vi "Main.vi"() -> ()   [LabVIEW 2021]
doc: "This template is for the Queued Message Handler design pattern.\n\nThe Event Handling Loop generates messages based on user interface actions.\n\nThe Message Handling Loop processes messages generated by the Event Handling Loop, or by other messages. The messages are string values, so new messages can be added easily to the Message Cases case structure in the Message Handling Loop. Each message cluster can also provide an optional value for Message Data, which is a variant that can be converted to whatever message-specific data is required."
uses:
  controls/UI Data.ctl
  support/Message Queue/Enqueue Message (Single).vi
  <vilib>/Analysis/3filter.llb/Butterworth Filter (DBL).vi
  <vilib>/Utility/error.llb/Error Cluster From Error Code.vi
  <vilib>/ErrorRing/Error Ring.xnode
  support/Message Queue/Message Queue.lvlib
  support/User Event - Stop/User Event - Stop.lvlib
  <vilib>/Analysis/NI_AALBase.lvlib
panel:
  in  "Engineering Mode":bool
  out "error out":errorcluster
  in  "Stop NanoJ":bool
  in  "Start NanoJ":bool
  out "Torque % of Max":dbl[](graph)
  in  "Read Torque":bool
  out "Motor Status":T1
  in  "Check Max Motor Current":bool
  out "Write":T2
  in  "Apply Speed":bool
  out "User Event":bool
  out "Actual Speed RPM":dbl(knob) scale=-110.0..110.0
  in  "Set Speed RPM":i32(knob) min=-60 max=60 scale=-60.0..60.0
  in  "Max Torque Nm":dbl=3.0 format="%.2f"
  out "Torque Nm":dbl
  out "Motor Current mA":dbl
  out "Max Motor Current mA":dbl
  out "Closed Loop Available":bool
  out "Motor Initialized":bool
  out "Torque\n%":dbl format="%.2f"
  in  "Halt Motor":bool
  in  "ComPort":refnum<visa-resource-name>="COM15"
  out "Program State":string
  in  "Start Motor":bool
  in  "Exit Program":bool
  # "<- Input max rated torque\nfor motor at Max Current Setting:"
  # "Current Motor Torque"
  # "Motor Current Draw"
  # "Set Speed Here \nthen click Apply\nto update Motor\nto new Velocity"
  # "Torque as percentage \nof Max Torque"
  # "Speed Value Read\nfrom Motor Memory"
  # "Restart the Motor Firmware\n(Hardware) Speed Controller\n(Disables LabVIEW Control)"
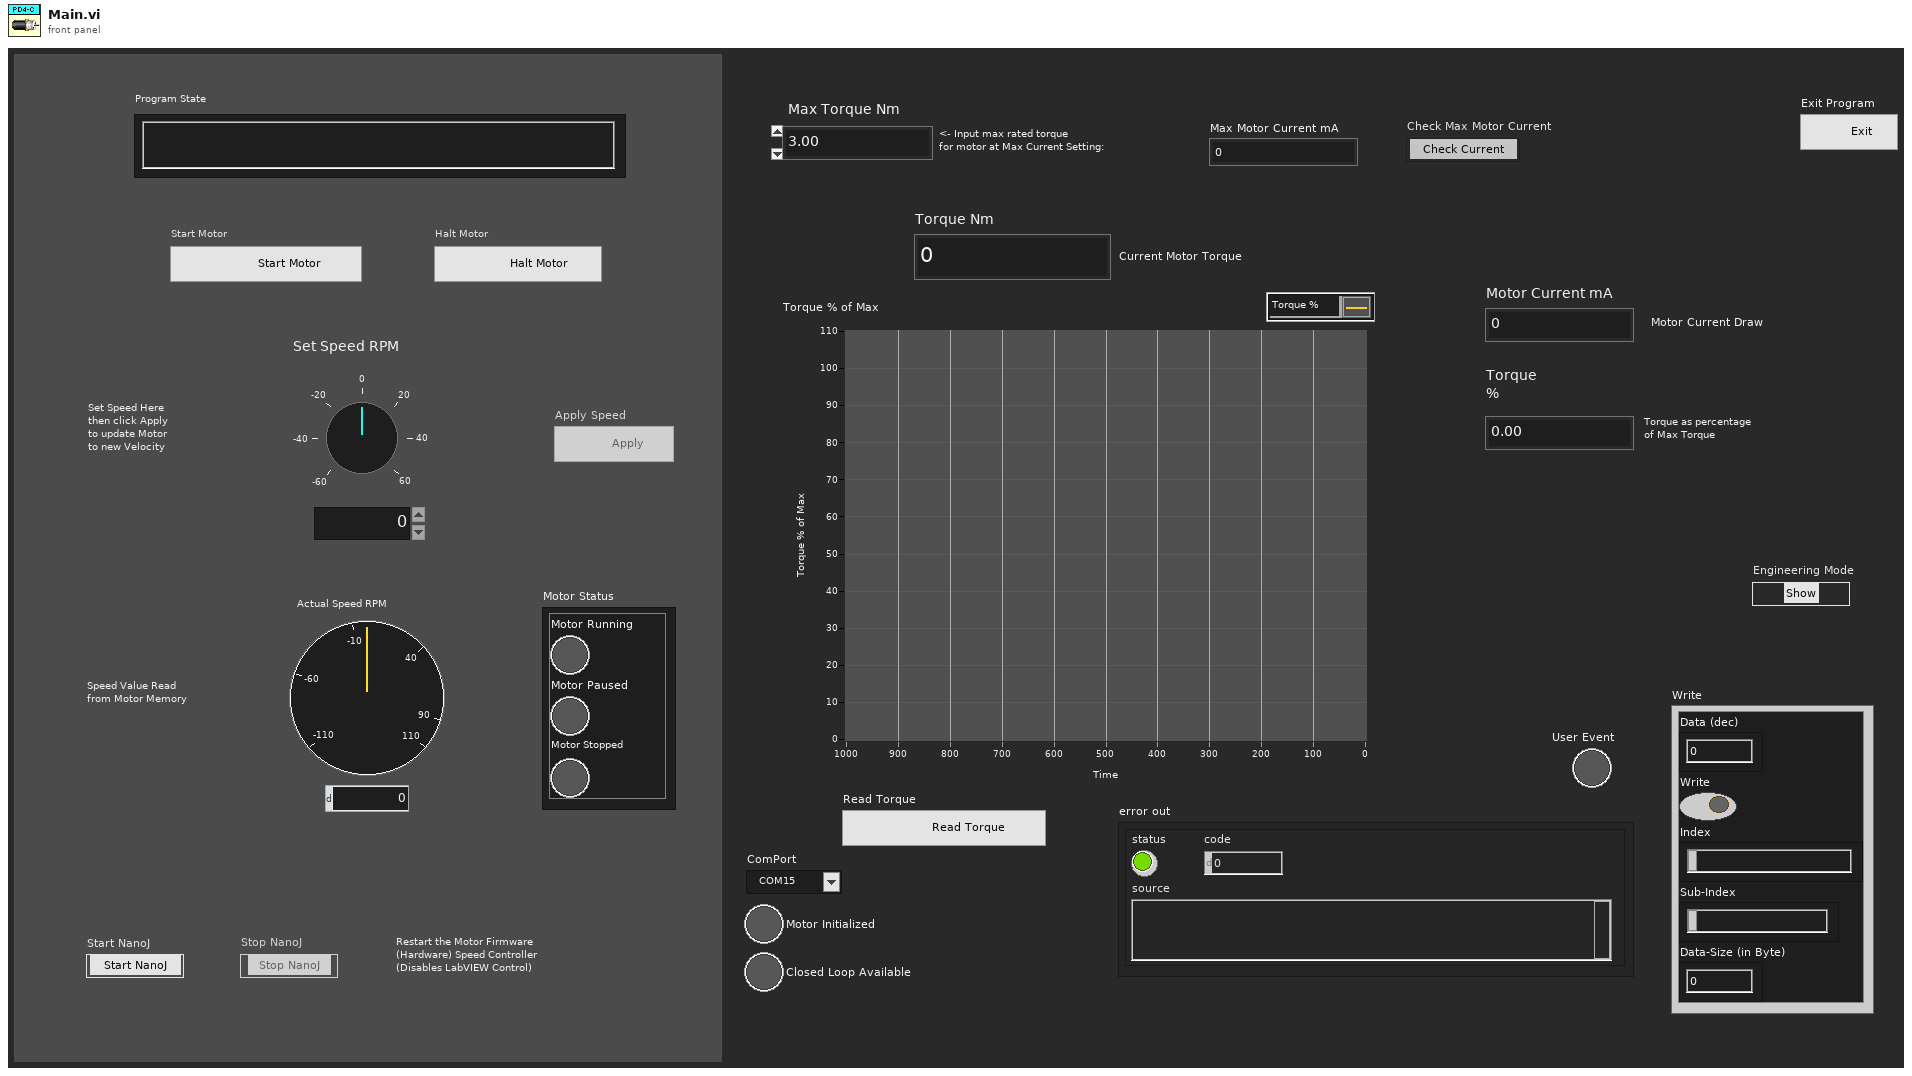
[diagram p1: front panel]
types:
  T1 = cluster{"Motor Running":bool, "Motor Paused":bool, "Motor Stopped":bool}
  T2 = cluster{"Data (dec)":i32, "Write":bool, "Index":string, "Sub-Index":string, "Data-Size (in Byte)":u8}
  T3 = typedef "UI Data.ctl" = cluster{"Data Display Ref":refnum<vi>, "Exit Button Ref":refnum<vi>, "VISA resource name":refnum<visa-resource-name>, "Write":cluster{"Data (dec)":i32, bool, "Index":string, "Sub-Index":string, "Data-Size (in Byte)":u8}, "Next State":string, "Data":i32}
  T4 = typedef "Message Queue.lvlib/All Message Queues.ctl" = cluster{"UI":refnum<queue>}
  T5 = enum8{"Enabled", "Disabled", "Disabled and Grayed Out"}
  T6 = cluster{"Motor Paused":bool, "Motor Running":bool, "Motor Stopped":bool}
  T7 = cluster{"Data (dec)":i32, bool, "Index":string, "Sub-Index":string, "Data-Size (in Byte)":u8}
  T8 = cluster{"Index":string, "Sub-Index":string, "Data-Size (in Byte)":u8, bool}
  T9 = cluster{"Motor Stopped":bool, "Motor Running":bool, "Motor Paused":bool}
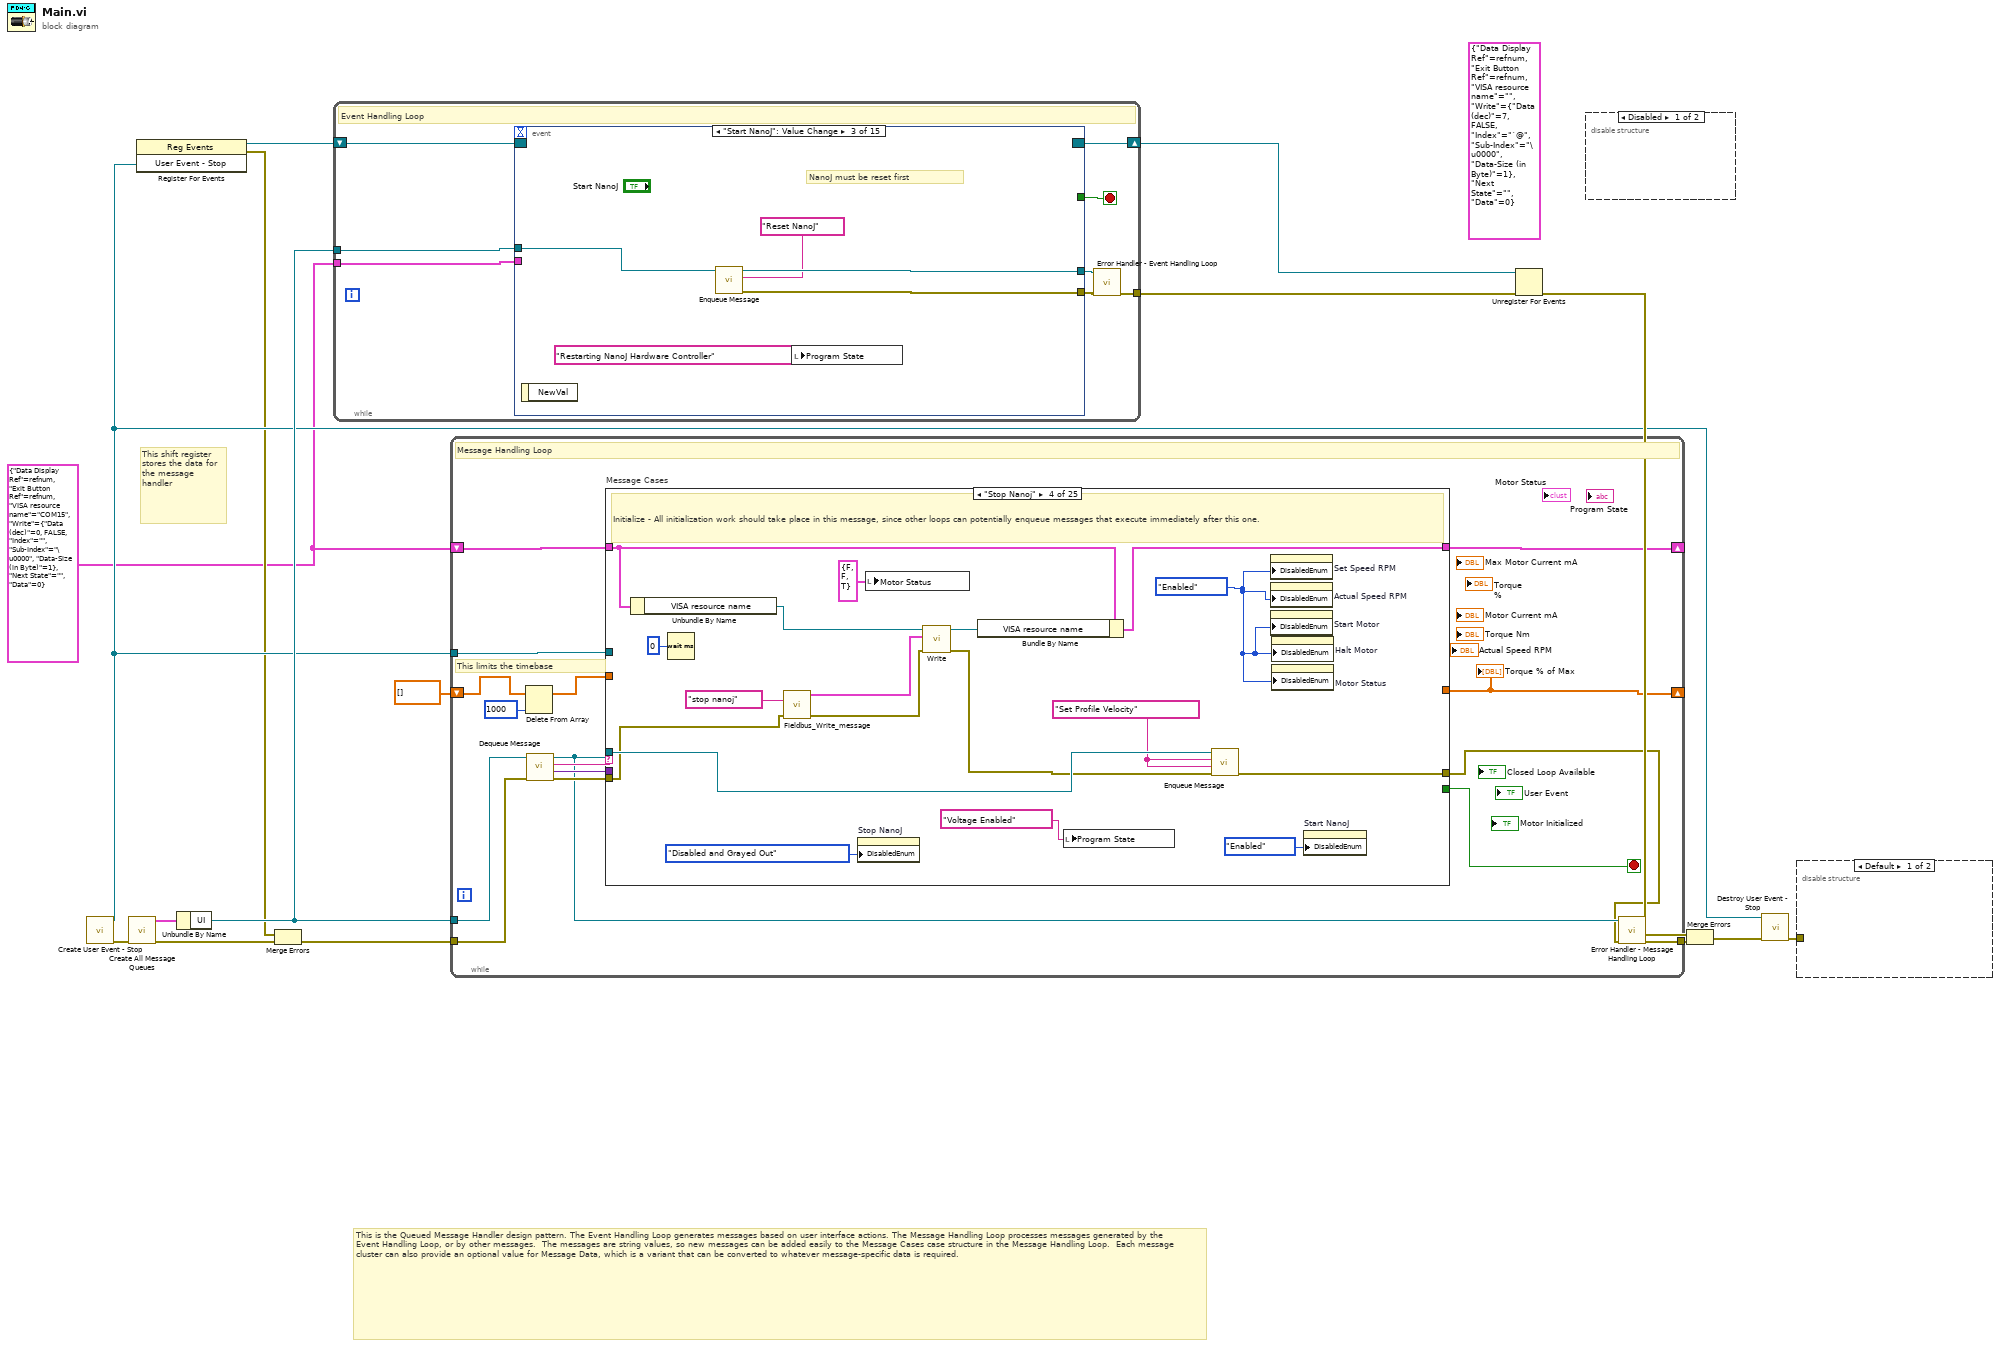
[diagram p0: block diagram]
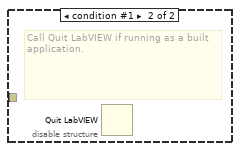
[diagram p3: hidden frame]
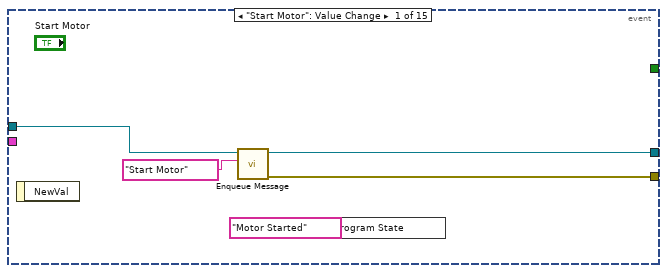
[diagram p4: hidden frame]
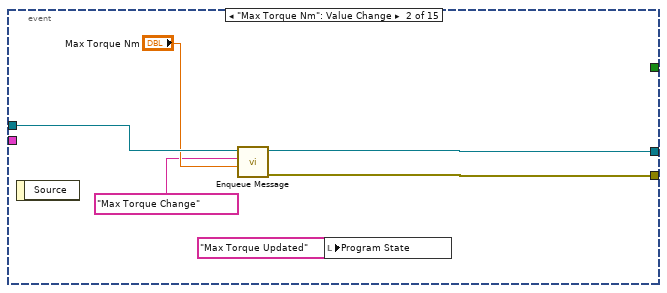
[diagram p5: hidden frame]
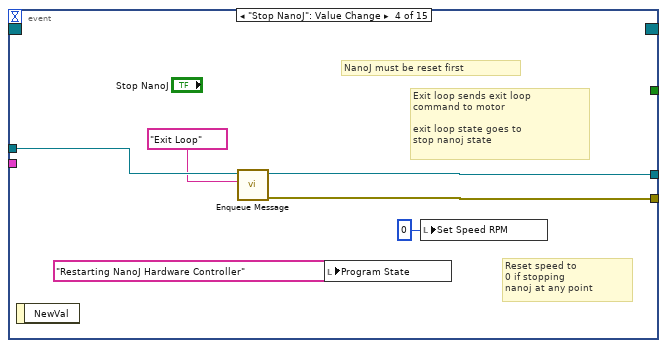
[diagram p6: hidden frame]
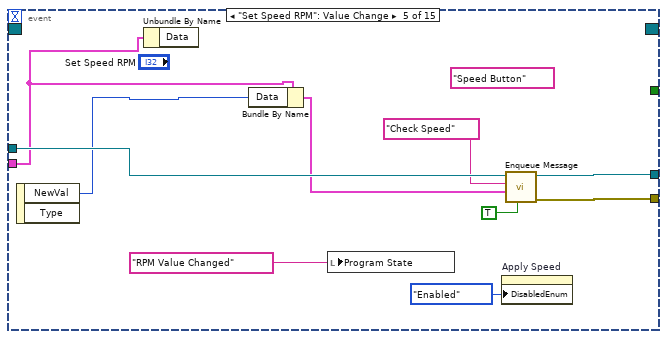
[diagram p7: hidden frame]
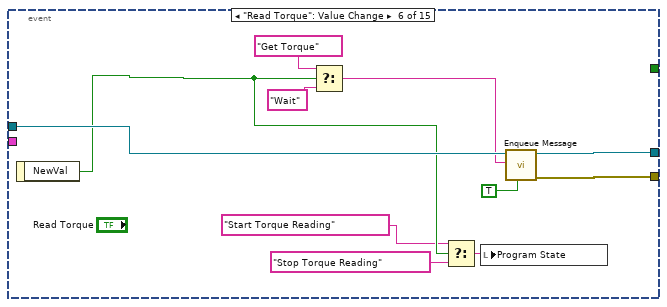
[diagram p8: hidden frame]
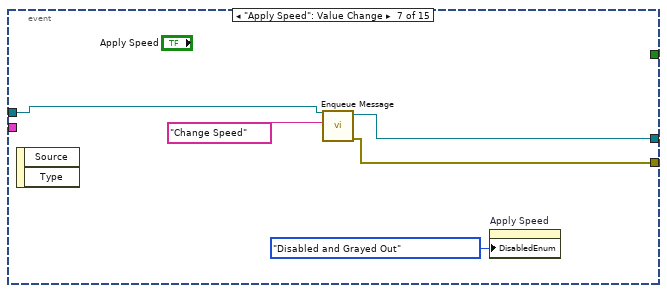
[diagram p9: hidden frame]
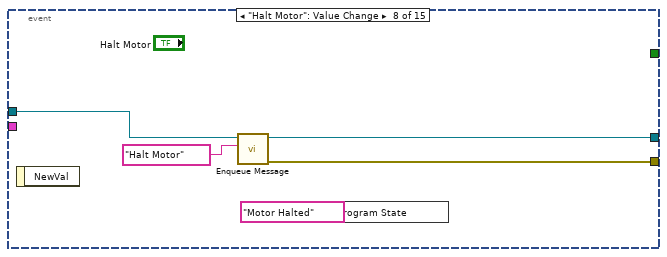
[diagram p10: hidden frame]
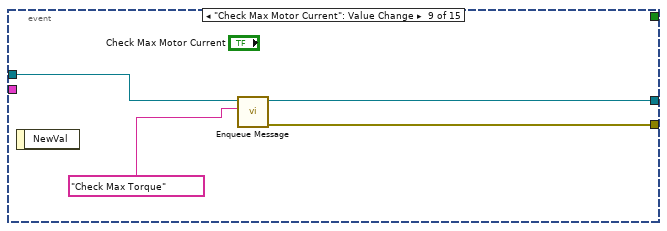
[diagram p11: hidden frame]
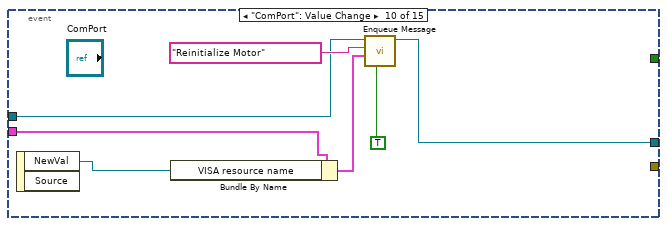
[diagram p12: hidden frame]
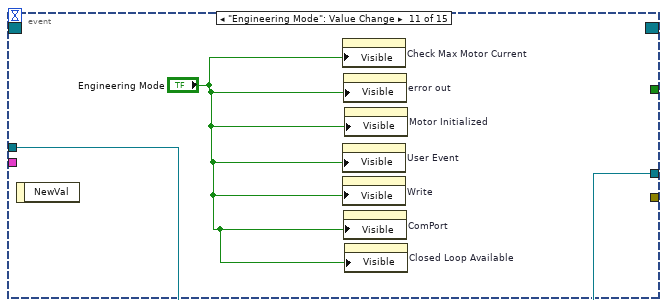
[diagram p13: hidden frame]
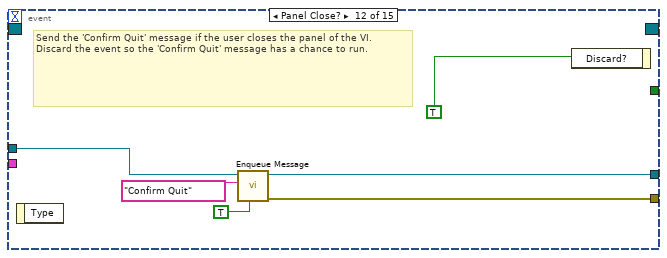
[diagram p14: hidden frame]
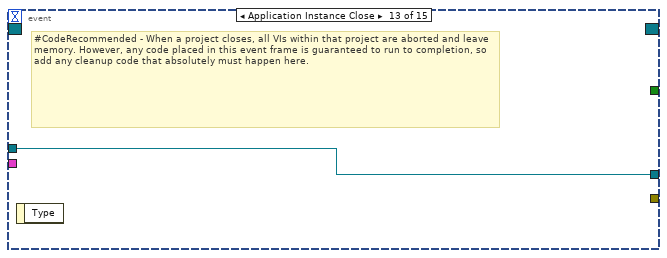
[diagram p15: hidden frame]
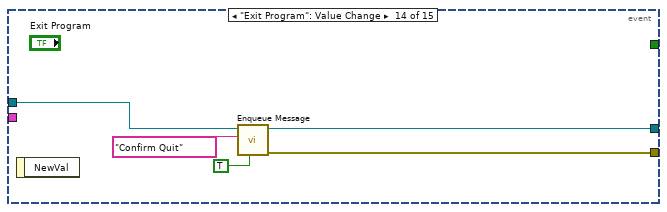
[diagram p16: hidden frame]
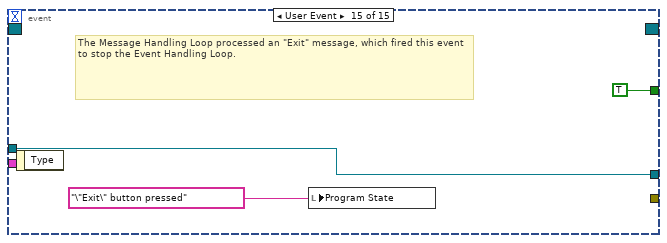
[diagram p17: hidden frame]
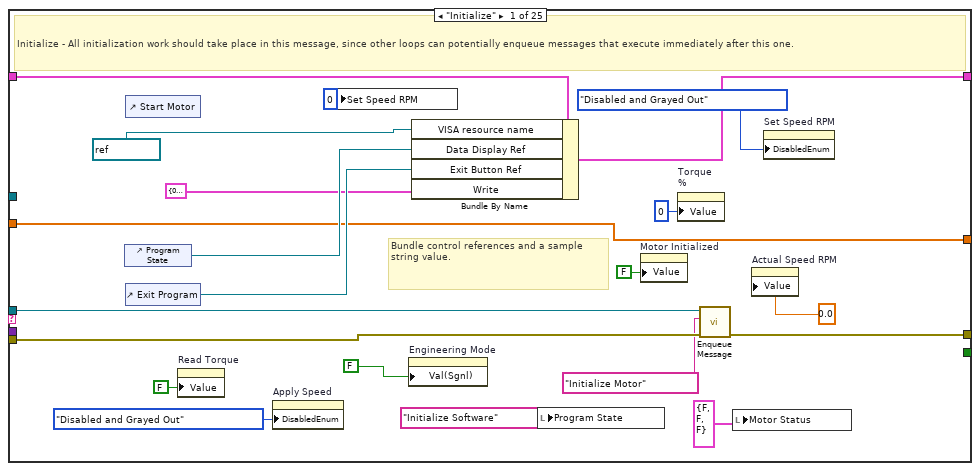
[diagram p18: hidden frame]
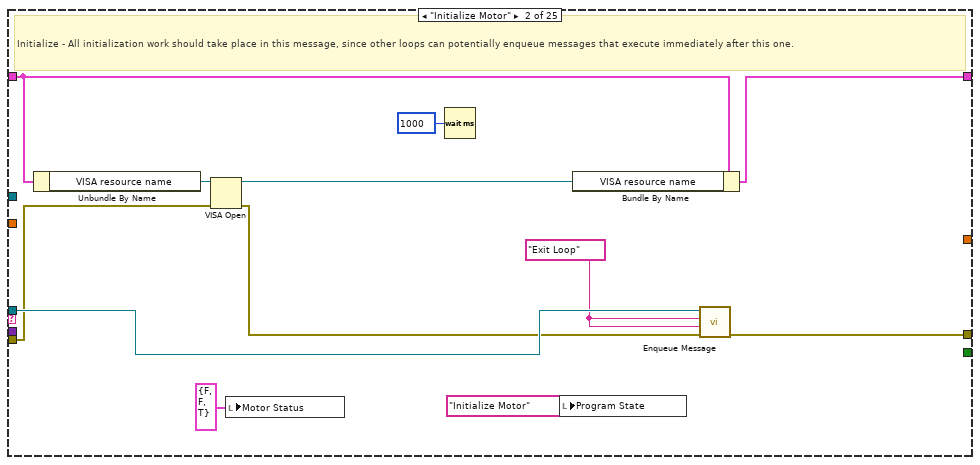
[diagram p19: hidden frame]
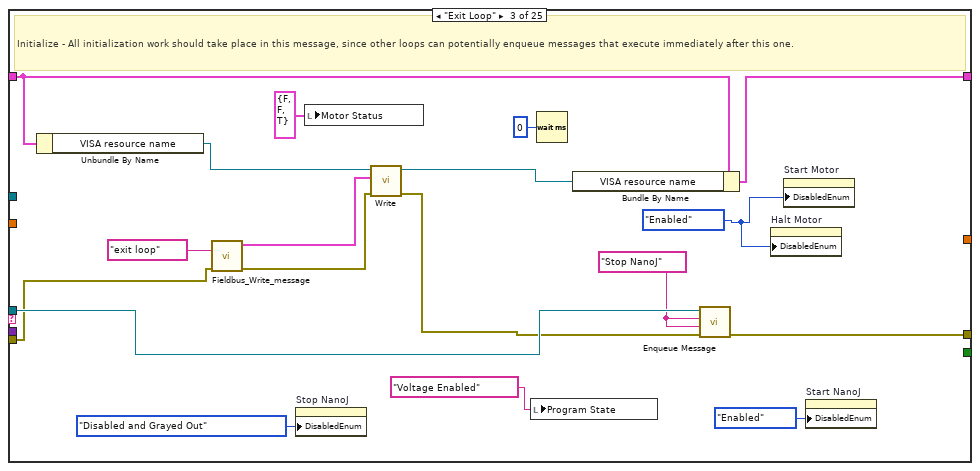
[diagram p20: hidden frame]
diagram:
  (unwired) T3 {"Data Display Ref"=refnum, "Exit Button Ref"=refnum, "VISA resource name"="", "Write"={"Data (dec)"=7, FALSE, "Index"="`@", "Sub-Index"="\u0000", "Data-Size (in Byte)"=1}, "Next State"="", "Data"=0} ("output cluster")
  w2 = T3 {"Data Display Ref"=refnum, "Exit Button Ref"=refnum, "VISA resource name"="COM15", "Write"={"Data (dec)"=0, FALSE, "Index"="", "Sub-Index"="\u0000", "Data-Size (in Byte)"=1}, "Next State"="", "Data"=0} ("Data Cluster")
  # "This is the Queued Message Handler design pattern. The Event Handling Loop generates messages based on user interface actions. The Message Handling Loop processes messages generated by the Event Handling Loop, or by other messages.  The messages are string values, so new messages can be added easily to the Message Cases case structure in the Message Handling Loop.  Each message cluster can also provide an optional value for Message Data, which is a variant that can be converted to whatever message-specific data is required."
  # "This shift register stores the data for the message handler"
  n1 = call "Create User Event - Stop.vi"() -> ("error out"=w12:errorcluster, "User Event - Stop"=w5:refnum<user-event>)  [unwired: 10 in]
  n2 = call "Create All Message Queues.vi"("error in (no error)"=w12) -> ("error out"=w16:errorcluster, "Message Queues out"=w15:T4)  [unwired: 9 in]
  n3 = register-events(w5) -> (reference out=w6:refnum<event-registration>, error out=w3:errorcluster)  [unwired: 2 in]
  n4 = Unbundle By Name "Unbundle By Name"(w15) -> ("UI"=w13:refnum<queue>)
  n5 = Merge Errors "Merge Errors"(w3, w16) -> (w4:errorcluster)
  n6 = while {
    tunnel: w13 -> [w24]
    shift-right: [w22] -> w9
    shift-left: w6 -> [w23]
    tunnel: [w18] -> w7
    tunnel: w2 -> [w17]
    stop <- w20 stop-if-true
    # "Event Handling Loop"
    n7 = event shown="[2] \"Start NanoJ\": Value Change" {
      selector: w23 -> [_ _ _ _ _ _ _ _ _ _ _ _ _ _ _]
      dyn-events: [_ _ _ _ _ _ _ _ _ _ _ _ _ _ _] -> w22
      timeout: _ -> [_ _ _ _ _ _ _ _ _ _ _ _ _ _ _]
      tunnel: [_ _ _ _ _ _ _ _ _ _ _ _ _ _ TRUE ("Discard?")] -> w20
      tunnel: w24 -> [w29 w35 w40 w46 w56 w67 w71 w77 w81 w87 w89 w95 w97 w102 w105]
      tunnel: [w26 w33 w38 w44 w54 w65 w69 w74 w78 _ _ w94 _ w101 _] -> w21
      tunnel: [w28 w34 w39 w45 w55 w66 w70 w76 w80 w86 w89 w93 w97 w100 w105] -> w19
      tunnel: w17 -> [_ _ _ _ w51 _ _ _ _ w82 _ _ _ _ _]
      event "Start Motor": Value Change {
        n8 = event-data() -> ()  [unwired: 1 in, 1 out]
        n9 = call-poly "Enqueue Message.vi"("Message"="Start Motor", "Message Queue"=w29) -> ("error out"=w26:errorcluster, "dup Message Queue"=w28:refnum<queue>)  [unwired: 8 in]
        n10 = local write "Program State"("Motor Started" ("State")) -> ()
      }
      event "Max Torque Nm": Value Change {
        n11 = event-data() -> ()  [unwired: 1 in, 1 out]
        n12 = call-poly "Enqueue Message.vi"("Message Data"="Max Torque Nm", "Message"="Max Torque Change", "Message Queue"=w35) -> ("error out"=w33:errorcluster, "dup Message Queue"=w34:refnum<queue>)  [unwired: 7 in]
        n13 = local write "Program State"("Max Torque Updated" ("State")) -> ()
      }
      event "Start NanoJ": Value Change {
        # "NanoJ must be reset first"
        n14 = event-data() -> ()  [unwired: 1 in, 1 out]
        n15 = call-poly "Enqueue Message.vi"("Message"="Reset NanoJ", "Message Queue"=w40) -> ("error out"=w38:errorcluster, "dup Message Queue"=w39:refnum<queue>)  [unwired: 8 in]
        n16 = local write "Program State"("Restarting NanoJ Hardware Controller" ("State")) -> ()
      }
      event "Stop NanoJ": Value Change {
        # "Reset speed to\n0 if stopping\nnanoj at any point"
        # "Exit loop sends exit loop\ncommand to motor\n\nexit loop state goes to\nstop nanoj state"
        # "NanoJ must be reset first"
        n17 = event-data() -> ()  [unwired: 1 in, 1 out]
        n18 = call-poly "Enqueue Message.vi"("Message"="Exit Loop", "Message Queue"=w46) -> ("error out"=w44:errorcluster, "dup Message Queue"=w45:refnum<queue>)  [unwired: 8 in]
        n19 = local write "Program State"("Restarting NanoJ Hardware Controller" ("State")) -> ()
        n20 = local write "Set Speed RPM"(0 ("Set Speed RPM")) -> ()
      }
      event "Set Speed RPM": Value Change {
        (unwired) "Speed Button" ("Message")
        n21 = event-data() -> ("NewVal"=w50:i32)  [unwired: 1 in, 1 out]
        n22 = Unbundle By Name(w51) -> ()  [unwired: 1 out]
        n23 = Bundle By Name(cluster=w51, "Data"=w50) -> (w53:T3)
        n24 = local write "Program State"("RPM Value Changed" ("State")) -> ()
        n25 = property on="Apply Speed" class="Bool"("DisabledEnum"=T5."Enabled" ("Disabled")) -> ()  [unwired: 2 in, 2 out]
        n26 = call-poly "Enqueue Message.vi"("Priority Message? (F)"=TRUE, "Message Data"=w53, "Message"="Check Speed", "Message Queue"=w56) -> ("error out"=w54:errorcluster, "dup Message Queue"=w55:refnum<queue>)  [unwired: 6 in]
      }
      event "Read Torque": Value Change {
        n27 = event-data() -> ("NewVal"=w63:bool)  [unwired: 1 in]
        n28 = Select(t="Get Torque" ("Message"), s=w63, f="Wait") -> (s? t:f=w58:string)
        n29 = Select(t="Start Torque Reading" ("State"), s=w63, f="Stop Torque Reading") -> (s? t:f=w57:string)
        n30 = local write "Program State"(w57) -> ()
        n31 = call-poly "Enqueue Message.vi"("Priority Message? (F)"=TRUE, "Message"=w58, "Message Queue"=w67) -> ("error out"=w65:errorcluster, "dup Message Queue"=w66:refnum<queue>)  [unwired: 7 in]
      }
      event "Apply Speed": Value Change {
        n32 = event-data() -> ()  [unwired: 1 in, 2 out]
        n33 = call-poly "Enqueue Message.vi"("Message"="Change Speed", "Message Queue"=w71) -> ("error out"=w69:errorcluster, "dup Message Queue"=w70:refnum<queue>)  [unwired: 8 in]
        n34 = property on="Apply Speed" class="Bool"("DisabledEnum"=T5."Disabled and Grayed Out" ("Disabled")) -> ()  [unwired: 2 in, 2 out]
      }
      event "Halt Motor": Value Change {
        n35 = event-data() -> ()  [unwired: 1 in, 1 out]
        n36 = call-poly "Enqueue Message.vi"("Message"="Halt Motor", "Message Queue"=w77) -> ("error out"=w74:errorcluster, "dup Message Queue"=w76:refnum<queue>)  [unwired: 8 in]
        n37 = local write "Program State"("Motor Halted" ("State")) -> ()
      }
      event "Check Max Motor Current": Value Change {
        n38 = event-data() -> ()  [unwired: 1 in, 1 out]
        n39 = call-poly "Enqueue Message.vi"("Message"="Check Max Torque", "Message Queue"=w81) -> ("error out"=w78:errorcluster, "dup Message Queue"=w80:refnum<queue>)  [unwired: 8 in]
      }
      event "ComPort": Value Change {
        n40 = event-data() -> ("NewVal"=w84:refnum<visa-resource-name>)  [unwired: 1 in, 1 out]
        n41 = Bundle By Name(cluster=w82, "VISA resource name"=w84) -> (w83:T3)
        n42 = call-poly "Enqueue Message.vi"("Priority Message? (F)"=TRUE, "Message Data"=w83, "Message"="Reinitialize Motor", "Message Queue"=w87) -> ("dup Message Queue"=w86:refnum<queue>)  [unwired: 6 in, 1 out]
      }
      event "Engineering Mode": Value Change {
        n43 = event-data() -> ()  [unwired: 1 in, 1 out]
        n44 = property on="Check Max Motor Current" class="Bool"("Visible"="Engineering Mode") -> ()  [unwired: 2 in, 2 out]
        n45 = property on="User Event" class="Bool (strict)"("Visible"="Engineering Mode") -> ()  [unwired: 2 in, 2 out]
        n46 = property on="Write" class="Clust (strict)"("Visible"="Engineering Mode") -> ()  [unwired: 2 in, 2 out]
        n47 = property on="error out" class="Clust (strict)"("Visible"="Engineering Mode") -> ()  [unwired: 2 in, 2 out]
        n48 = property on="ComPort" class="VISAName"("Visible"="Engineering Mode") -> ()  [unwired: 2 in, 2 out]
        n49 = property on="Motor Initialized" class="Bool (strict)"("Visible"="Engineering Mode") -> ()  [unwired: 2 in, 2 out]
        n50 = property on="Closed Loop Available" class="Bool (strict)"("Visible"="Engineering Mode") -> ()  [unwired: 2 in, 2 out]
      }
      event Panel Close? {
        # "Send the 'Confirm Quit' message if the user closes the panel of the VI. Discard the event so the 'Confirm Quit' message has a chance to run."
        n51 = event-data() -> ()  [unwired: 1 in, 1 out]
        n52 = call-poly "Enqueue Message.vi"("Priority Message? (F)"=TRUE, "Message"="Confirm Quit", "Message Queue"=w95) -> ("error out"=w94:errorcluster, "dup Message Queue"=w93:refnum<queue>)  [unwired: 7 in]
        n53 = event-data("Discard?"=TRUE) -> ()  [unwired: 1 in, 1 out]
      }
      event Application Instance Close {
        # "#CodeRecommended - When a project closes, all VIs within that project are aborted and leave memory. However, any code placed in this event frame is guaranteed to run to completion, so add any cleanup code that absolutely must happen here."
        n54 = event-data() -> ()  [unwired: 1 in, 1 out]
      }
      event "Exit Program": Value Change {
        n55 = event-data() -> ()  [unwired: 1 in, 1 out]
        n56 = call-poly "Enqueue Message.vi"("Priority Message? (F)"=TRUE, "Message"="Confirm Quit", "Message Queue"=w102) -> ("error out"=w101:errorcluster, "dup Message Queue"=w100:refnum<queue>)  [unwired: 7 in]
      }
      event User Event {
        # "The Message Handling Loop processed an \"Exit\" message, which fired this event to stop the Event Handling Loop."
        n57 = event-data() -> ()  [unwired: 1 in, 1 out]
        n58 = local write "Program State"("\"Exit\" button pressed" ("VI Stopped")) -> ()
      }
    }
    n59 = call "Error Handler - Event Handling Loop.vi"("error in (no error)"=w21, "Message Queue"=w19) -> ("dup error in"=w18:errorcluster)  [unwired: 8 in, 1 out]
  }
  n60 = while {
    tunnel: w13 -> [w114]
    shift-right: [w120] -> _
    shift-left: w2 -> [w121]
    tunnel: w5 -> [w119]
    tunnel: w4 -> [w118]
    tunnel: [w112] -> w14
    shift-right: [w111] -> _
    shift-left: dbl[] [] -> [w107]
    stop <- w109 stop-if-true
    # "This limits the timebase"
    # "Message Handling Loop"
    n61 = Delete From Array(array=w107, index=1000) -> (array with subset deleted=w106:dbl[])  [unwired: 1 in, 1 out]
    n62 = call "Dequeue Message.vi"("error in (no error)"=w118, "Message Queue"=w114) -> ("error out"=w117:errorcluster, "Message Data"=w115:variant, "Message"=w116:string, "dup Message Queue"=w113:refnum<queue>)  [unwired: 6 in]
    n63 = case "Message Cases" shown="\"Stop Nanoj\"" w116 {
      selector: w116 -> [_ _ _ _ _ _ _ _ _ _ _ _ _ _ _ _ _ _ _ _ _ _ _ _ w480]
      tunnel: w113 -> [w130 w153 w171 w189 w203 w217 w235 w252 w266 w283 w300 w322 w344 w359 w363 w379 _ w398 w420 _ _ w449 w467 w478 _]
      tunnel: w117 -> [w141 w151 w161 w179 w192 w206 w224 w241 w256 w280 w297 w319 w341 w347 w361 w380 w385 w388 w417 w426 w435 w437 w456 w472 _]
      tunnel: [w142 w154 w172 w190 w204 w218 w236 w253 w267 w284 w301 w323 w345 w360 w375 w377 w385 w399 w421 w427 w429 w451 w464 w479 w481] -> w110
      tunnel: w121 -> [w140 w150 w170 w188 w202 w216 w234 w251 w265 w282 w299 w321 w343 w358 w365 w381 w386 w397 w419 w428 w434 w441 w457 w473 w482]
      tunnel: [w139 w149 w169 w187 w201 w215 w233 w250 w264 w281 w298 w320 w342 w357 w374 w381 w386 w396 w418 w428 w434 w440 w457 w477 w482] -> w120
      tunnel: [_ _ _ _ _ _ _ _ _ _ _ _ _ _ _ _ _ _ _ _ _ _ TRUE _ _] -> w109
      tunnel: w115 -> [_ _ _ _ _ _ _ _ _ _ _ _ _ _ _ _ _ _ _ w425 w433 _ w459 w468 _]
      tunnel: w119 -> [_ _ _ _ _ _ _ _ _ _ _ _ _ _ _ _ _ _ _ _ _ _ w463 _ _]
      tunnel: [w125 _ _ _ _ _ _ _ _ _ _ _ _ _ _ _ _ _ w400 _ _ _ _ _ _] -> w111
      tunnel: w106 -> [w125 _ _ _ _ _ _ _ _ _ _ _ _ _ _ _ _ _ w408 _ _ _ _ _ _]
      frame "Initialize" {
        # "Bundle control references and a sample string value."
        # "Initialize - All initialization work should take place in this message, since other loops can potentially enqueue messages that execute immediately after this one."
        n64 = control-ref of="Program State"() -> (w138:refnum<vi>)
        n65 = control-ref of="Start Motor"() -> ()  [unwired: 1 out]
        n66 = control-ref of="Exit Program"() -> (w137:refnum<vi>)
        n67 = property on="Read Torque" class="Bool (strict)"("Value"=FALSE ("Read Torque")) -> ()  [unwired: 2 in, 2 out]
        n68 = property on="Apply Speed" class="Bool"("DisabledEnum"=T5."Disabled and Grayed Out" ("Disabled")) -> ()  [unwired: 2 in, 2 out]
        n69 = local write "Set Speed RPM"(0 ("Speed RPM")) -> ()
        n70 = property on="Engineering Mode" class="Bool (strict)"("Val(Sgnl)"=FALSE ("Engineering Mode")) -> ()  [unwired: 2 in, 2 out]
        n71 = Bundle By Name "Bundle By Name"(cluster=w140, "VISA resource name"=refnum<visa-resource-name> "COM15", "Data Display Ref"=w138, "Exit Button Ref"=w137, "Write"=T7 {"Data (dec)"=0, FALSE, "Index"="", "Sub-Index"="", "Data-Size (in Byte)"=0}) -> (w139:T3)
        n72 = local write "Program State"("Initialize Software" ("State")) -> ()
        n73 = property on="Motor Initialized" class="Bool (strict)"("Value"=FALSE ("Motor Initialized")) -> ()  [unwired: 2 in, 2 out]
        n74 = property on="Torque\n%" class="DigNum (strict)"("Value"=0 ("Torque\n%")) -> ()  [unwired: 2 in, 2 out]
        n75 = call-poly "Enqueue Message.vi"("error in (no error)"=w141, "Message"="Initialize Motor", "Message Queue"=w130) -> ("error out"=w142:errorcluster)  [unwired: 7 in, 1 out]
        n76 = local write "Motor Status"(T6 {"Motor Paused"=FALSE, "Motor Running"=FALSE, "Motor Stopped"=FALSE} ("Motor Status")) -> ()
        n77 = property on="Actual Speed RPM" class="Knob (strict)"("Value"=0.0 ("Speed RPM")) -> ()  [unwired: 2 in, 2 out]
        n78 = property on="Set Speed RPM" class="Knob (strict)"("DisabledEnum"=T5."Disabled and Grayed Out" ("Disabled")) -> ()  [unwired: 2 in, 2 out]
      }
      frame "Initialize Motor" {
        w146 = "Exit Loop" ("Message")
        # "Initialize - All initialization work should take place in this message, since other loops can potentially enqueue messages that execute immediately after this one."
        n79 = Unbundle By Name(w150) -> ("VISA resource name"=w152:refnum<visa-resource-name>)
        n80 = VISA Open(error in (no error)=w151, VISA resource name=w152) -> (VISA resource name=w148:refnum<visa-resource-name>, error out=w147:errorcluster)  [unwired: 3 in]
        n81 = local write "Motor Status"(T1 {"Motor Running"=FALSE, "Motor Paused"=FALSE, "Motor Stopped"=TRUE} ("Motor Status")) -> ()
        n82 = Wait (ms)(milliseconds to wait=u32 1000) -> ()  [unwired: 1 out]
        n83 = local write "Program State"("Initialize Motor" ("State")) -> ()
        n84 = Bundle By Name(cluster=w150, "VISA resource name"=w148) -> (w149:T3)
        n85 = call-poly "Enqueue Message.vi"("error in (no error)"=w147, "Message Data"=w146, "Message"=w146, "Message Queue"=w153) -> ("error out"=w154:errorcluster)  [unwired: 6 in, 1 out]
      }
      frame "Exit Loop" {
        w158 = T5."Enabled" ("Disabled")
        w167 = "Stop NanoJ" ("Message")
        # "Initialize - All initialization work should take place in this message, since other loops can potentially enqueue messages that execute immediately after this one."
        n86 = Unbundle By Name(w170) -> ("VISA resource name"=w166:refnum<visa-resource-name>)
        n87 = call "Fieldbus_Write_message.vi"("error in"=w161, "Message"="exit loop") -> ("error output"=w160:errorcluster, "Write"=w165:T2)  [unwired: 8 in]
        n88 = property on="Stop NanoJ" class="Bool"("DisabledEnum"=T5."Disabled and Grayed Out" ("Disabled")) -> ()  [unwired: 2 in, 2 out]
        n89 = local write "Motor Status"(T1 {"Motor Running"=FALSE, "Motor Paused"=FALSE, "Motor Stopped"=TRUE} ("Motor Status")) -> ()
        n90 = call "Write.vi"("error in"=w160, "Write"=w165, "ComPort In"=w166) -> ("error out"=w159:errorcluster, "ComPort Out"=w168:refnum<visa-resource-name>)  [unwired: 7 in]
        n91 = local write "Program State"("Voltage Enabled" ("State")) -> ()
        n92 = Wait (ms)(milliseconds to wait=u32 0) -> ()  [unwired: 1 out]
        n93 = Bundle By Name(cluster=w170, "VISA resource name"=w168) -> (w169:T3)
        n94 = call-poly "Enqueue Message.vi"("error in (no error)"=w159, "Message Data"=w167, "Message"=w167, "Message Queue"=w171) -> ("error out"=w172:errorcluster)  [unwired: 6 in, 1 out]
        n95 = property on="Halt Motor" class="Bool"("DisabledEnum"=w158) -> ()  [unwired: 2 in, 2 out]
        n96 = property on="Start Motor" class="Bool"("DisabledEnum"=w158) -> ()  [unwired: 2 in, 2 out]
        n97 = property on="Start NanoJ" class="Bool"("DisabledEnum"=T5."Enabled" ("Disabled")) -> ()  [unwired: 2 in, 2 out]
      }
      frame "Stop Nanoj" {
        w173 = T5."Enabled" ("Disabled")
        w185 = "Set Profile Velocity" ("Message")
        # "Initialize - All initialization work should take place in this message, since other loops can potentially enqueue messages that execute immediately after this one."
        n98 = Unbundle By Name(w188) -> ("VISA resource name"=w184:refnum<visa-resource-name>)
        n99 = Wait (ms)(milliseconds to wait=u32 0) -> ()  [unwired: 1 out]
        n100 = call "Fieldbus_Write_message.vi"("error in"=w179, "Message"="stop nanoj") -> ("error output"=w178:errorcluster, "Write"=w183:T2)  [unwired: 8 in]
        n101 = property on="Stop NanoJ" class="Bool"("DisabledEnum"=T5."Disabled and Grayed Out" ("Disabled")) -> ()  [unwired: 2 in, 2 out]
        n102 = local write "Motor Status"(T1 {"Motor Running"=FALSE, "Motor Paused"=FALSE, "Motor Stopped"=TRUE} ("Motor Status")) -> ()
        n103 = call "Write.vi"("error in"=w178, "Write"=w183, "ComPort In"=w184) -> ("error out"=w177:errorcluster, "ComPort Out"=w186:refnum<visa-resource-name>)  [unwired: 7 in]
        n104 = Bundle By Name(cluster=w188, "VISA resource name"=w186) -> (w187:T3)
        n105 = local write "Program State"("Voltage Enabled" ("State")) -> ()
        n106 = call-poly "Enqueue Message.vi"("error in (no error)"=w177, "Message Data"=w185, "Message"=w185, "Message Queue"=w189) -> ("error out"=w190:errorcluster)  [unwired: 6 in, 1 out]
        n107 = property on="Set Speed RPM" class="Knob (strict)"("DisabledEnum"=w173) -> ()  [unwired: 2 in, 2 out]
        n108 = property on="Actual Speed RPM" class="Knob (strict)"("DisabledEnum"=w173) -> ()  [unwired: 2 in, 2 out]
        n109 = property on="Start Motor" class="Bool"("DisabledEnum"=w173) -> ()  [unwired: 2 in, 2 out]
        n110 = property on="Halt Motor" class="Bool"("DisabledEnum"=w173) -> ()  [unwired: 2 in, 2 out]
        n111 = property on="Motor Status" class="Clust (strict)"("DisabledEnum"=w173) -> ()  [unwired: 2 in, 2 out]
        n112 = property on="Start NanoJ" class="Bool"("DisabledEnum"=T5."Enabled" ("Disabled")) -> ()  [unwired: 2 in, 2 out]
      }
      frame "Set Profile Velocity" {
        w198 = "Change Speed" ("Message")
        # "Initialize - All initialization work should take place in this message, since other loops can potentially enqueue messages that execute immediately after this one."
        n113 = Unbundle By Name(w202) -> ("VISA resource name"=w197:refnum<visa-resource-name>)  [unwired: 1 out]
        n114 = call "Fieldbus_Write_message.vi"("error in"=w192, "Message"="profile velocity") -> ("error output"=w191:errorcluster, "Write"=w196:T2)  [unwired: 8 in]
        n115 = call "Write.vi"("error in"=w191, "Write"=w196, "ComPort In"=w197) -> ("error out"=w199:errorcluster, "ComPort Out"=w200:refnum<visa-resource-name>)  [unwired: 7 in]
        n116 = local write "Program State"("Voltage Enabled" ("State")) -> ()
        n117 = Wait (ms)(milliseconds to wait=u32 500) -> ()  [unwired: 1 out]
        n118 = Bundle By Name(cluster=w202, "VISA resource name"=w200) -> (w201:T3)
        n119 = call-poly "Enqueue Message.vi"("error in (no error)"=w199, "Message Data"=w198, "Message"=w198, "Message Queue"=w203) -> ("error out"=w204:errorcluster)  [unwired: 6 in, 1 out]
      }
      frame "Enable Voltage" {
        w212 = "Set Closed Loop" ("Message")
        # "Initialize - All initialization work should take place in this message, since other loops can potentially enqueue messages that execute immediately after this one."
        n120 = Unbundle By Name(w216) -> ("VISA resource name"=w211:refnum<visa-resource-name>)  [unwired: 1 out]
        n121 = call "Fieldbus_Write_message.vi"("error in"=w206, "Message"="enable voltage") -> ("error output"=w205:errorcluster, "Write"=w210:T2)  [unwired: 8 in]
        n122 = call "Write.vi"("error in"=w205, "Write"=w210, "ComPort In"=w211) -> ("error out"=w213:errorcluster, "ComPort Out"=w214:refnum<visa-resource-name>)  [unwired: 7 in]
        n123 = local write "Program State"("Voltage Enabled" ("State")) -> ()
        n124 = Wait (ms)(milliseconds to wait=u32 1000) -> ()  [unwired: 1 out]
        n125 = Bundle By Name(cluster=w216, "VISA resource name"=w214) -> (w215:T3)
        n126 = call-poly "Enqueue Message.vi"("error in (no error)"=w213, "Message Data"=w212, "Message"=w212, "Message Queue"=w217) -> ("error out"=w218:errorcluster)  [unwired: 6 in, 1 out]
      }
      frame "Start NanoJ" {
        w230 = "Wait" ("Message")
        # "Initialize - All initialization work should take place in this message, since other loops can potentially enqueue messages that execute immediately after this one."
        n127 = Unbundle By Name(w234) -> ("VISA resource name"=w229:refnum<visa-resource-name>)  [unwired: 1 out]
        n128 = local write "Motor Status"(T1 {"Motor Running"=TRUE, "Motor Paused"=TRUE, "Motor Stopped"=TRUE} ("Motor Status")) -> ()
        n129 = call "Fieldbus_Write_message.vi"("error in"=w224, "Message"="start nanoj") -> ("error output"=w223:errorcluster, "Write"=w228:T2)  [unwired: 8 in]
        n130 = call "Write.vi"("error in"=w223, "Write"=w228, "ComPort In"=w229) -> ("error out"=w231:errorcluster, "ComPort Out"=w232:refnum<visa-resource-name>)  [unwired: 7 in]
        n131 = local write "Program State"("NanoJ Program Active" ("State")) -> ()
        n132 = Wait (ms)(milliseconds to wait=u32 1000) -> ()  [unwired: 1 out]
        n133 = Bundle By Name(cluster=w234, "VISA resource name"=w232) -> (w233:T3)
        n134 = call-poly "Enqueue Message.vi"("error in (no error)"=w231, "Message Data"=w230, "Message"=w230, "Message Queue"=w235) -> ("error out"=w236:errorcluster)  [unwired: 6 in, 1 out]
        n135 = local write "Motor Initialized"(FALSE ("Motor Initialized")) -> ()
        n136 = property on="Stop NanoJ" class="Bool"("DisabledEnum"=T5."Enabled" ("Disabled")) -> ()  [unwired: 2 in, 2 out]
        n137 = property on="Start NanoJ" class="Bool"("DisabledEnum"=T5."Disabled and Grayed Out" ("Disabled")) -> ()  [unwired: 2 in, 2 out]
      }
      frame "Reset NanoJ" {
        w237 = T5."Disabled and Grayed Out" ("Disabled")
        w247 = "Start NanoJ" ("Message")
        # "Initialize - All initialization work should take place in this message, since other loops can potentially enqueue messages that execute immediately after this one."
        n138 = Unbundle By Name(w251) -> ("VISA resource name"=w246:refnum<visa-resource-name>)  [unwired: 1 out]
        n139 = local write "Motor Status"(T1 {"Motor Running"=TRUE, "Motor Paused"=TRUE, "Motor Stopped"=TRUE} ("Motor Status")) -> ()
        n140 = call "Fieldbus_Write_message.vi"("error in"=w241, "Message"="reset nanoj") -> ("error output"=w240:errorcluster, "Write"=w245:T2)  [unwired: 8 in]
        n141 = call "Write.vi"("error in"=w240, "Write"=w245, "ComPort In"=w246) -> ("error out"=w248:errorcluster, "ComPort Out"=w249:refnum<visa-resource-name>)  [unwired: 7 in]
        n142 = local write "Program State"("NanoJ Program Active" ("State")) -> ()
        n143 = Wait (ms)(milliseconds to wait=u32 1000) -> ()  [unwired: 1 out]
        n144 = Bundle By Name(cluster=w251, "VISA resource name"=w249) -> (w250:T3)
        n145 = local write "Motor Initialized"(FALSE ("Motor Initialized")) -> ()
        n146 = call-poly "Enqueue Message.vi"("error in (no error)"=w248, "Message Data"=w247, "Message"=w247, "Message Queue"=w252) -> ("error out"=w253:errorcluster)  [unwired: 6 in, 1 out]
        n147 = property on="Start Motor" class="Bool"("DisabledEnum"=w237) -> ()  [unwired: 2 in, 2 out]
        n148 = property on="Halt Motor" class="Bool"("DisabledEnum"=w237) -> ()  [unwired: 2 in, 2 out]
        n149 = property on="Set Speed RPM" class="Knob (strict)"("DisabledEnum"=w237) -> ()  [unwired: 2 in, 2 out]
        n150 = property on="Motor Status" class="Clust (strict)"("DisabledEnum"=w237) -> ()  [unwired: 2 in, 2 out]
        n151 = property on="Actual Speed RPM" class="Knob (strict)"("DisabledEnum"=w237) -> ()  [unwired: 2 in, 2 out]
      }
      frame "Set Closed Loop" {
        w261 = "Check Closed Loop" ("Message")
        # "Initialize - All initialization work should take place in this message, since other loops can potentially enqueue messages that execute immediately after this one."
        n152 = Unbundle By Name(w265) -> ("VISA resource name"=w260:refnum<visa-resource-name>)  [unwired: 1 out]
        n153 = call "Fieldbus_Write_message.vi"("error in"=w256, "Message"="closed loop mode") -> ("error output"=w255:errorcluster, "Write"=w259:T2)  [unwired: 8 in]
        n154 = property on="Set Speed RPM" class="Knob (strict)"("DisabledEnum"=T5."Enabled" ("Disabled")) -> ()  [unwired: 2 in, 2 out]
        n155 = call "Write.vi"("error in"=w255, "Write"=w259, "ComPort In"=w260) -> ("error out"=w262:errorcluster, "ComPort Out"=w263:refnum<visa-resource-name>)  [unwired: 7 in]
        n156 = Bundle By Name(cluster=w265, "VISA resource name"=w263) -> (w264:T3)
        n157 = local write "Program State"("Setting Closed Loop Mode" ("State")) -> ()
        n158 = call-poly "Enqueue Message.vi"("error in (no error)"=w262, "Message Data"=w261, "Message"=w261, "Message Queue"=w266) -> ("error out"=w267:errorcluster)  [unwired: 6 in, 1 out]
      }
      frame "Check Closed Loop" {
        (unwired) "torque" ("Message")
        # "Initialize - All initialization work should take place in this message, since other loops can potentially enqueue messages that execute immediately after this one."
        n159 = Unbundle By Name(w282) -> ("VISA resource name"=w277:refnum<visa-resource-name>)
        n160 = local read "Motor Status"() -> (w271:T1)
        n161 = Unbundle By Name(w271) -> ("Motor Stopped"=w268:bool)  [unwired: 2 out]
        n162 = call "Read.vi"("error out"=w280, "Read"=T8 {"Index"="`A", "Sub-Index"="\u0000", "Data-Size (in Byte)"=2, TRUE}, "ComPort In"=w277) -> ("error out 2"=w279:errorcluster, "Answer"=w275:i32, "ComPort Out"=w276:refnum<visa-resource-name>)  [unwired: 6 in]
        n163 = Bundle By Name(cluster=w282, "VISA resource name"=w276) -> (w281:T3)
        n164 = Select(t="Check Max Torque" ("f"), s=w268, f="Wait" ("Message")) -> (s? t:f=w274:string)
        n165 = call "Check Closed Loop.vi"("Answer"=w275) -> ("Bit 0"=w273:bool)  [unwired: 9 in, 1 out]
        n166 = local write "Program State"("Checking Closed Loop" ("State")) -> ()
        n167 = call-poly "Enqueue Message.vi"("error in (no error)"=w279, "Message"=w274, "Message Queue"=w283) -> ("error out"=w284:errorcluster)  [unwired: 7 in, 1 out]
        n168 = property on="Closed Loop Available" class="Bool (strict)"("Value"=w273) -> ()  [unwired: 2 in, 2 out]
      }
      frame "Check Max Torque" {
        (unwired) "torque" ("Message")
        # "Initialize - All initialization work should take place in this message, since other loops can potentially enqueue messages that execute immediately after this one."
        n169 = Unbundle By Name(w299) -> ("VISA resource name"=w294:refnum<visa-resource-name>)
        n170 = local read "Motor Status"() -> (w289:T1)
        n171 = for {
          N: 2 -> [_]
          tunnel: T8 {"Index"=" 1", "Sub-Index"="\u0000", "Data-Size (in Byte)"=4, TRUE} ("Read") -> [w305]
          tunnel: [w302] -> w291
          shift-right: [w306] -> w296
          shift-left: w297 -> [w307]
          shift-right: [w303] -> w293
          shift-left: w294 -> [w304]
          n172 = call "Read.vi"("error out"=w307, "Read"=w305, "ComPort In"=w304) -> ("error out 2"=w306:errorcluster, "Answer"=w302:i32, "ComPort Out"=w303:refnum<visa-resource-name>)  [unwired: 6 in]
        }
        n173 = Unbundle By Name(w289) -> ("Motor Stopped"=w288:bool)  [unwired: 2 out]
        n174 = property on="Motor Initialized" class="Bool (strict)" props=["Value"]() -> ()  [unwired: 2 in, 3 out]
        n175 = property on="Max Motor Current mA" class="DigNum (strict)"("Value"=w291) -> ()  [unwired: 2 in, 2 out]
        n176 = Bundle By Name(cluster=w299, "VISA resource name"=w293) -> (w298:T3)
        n177 = Select(t="Halt Motor" ("f"), s=w288, f="Wait" ("Message")) -> (s? t:f=w292:string)
        n178 = call-poly "Enqueue Message.vi"("error in (no error)"=w296, "Message"=w292, "Message Queue"=w300) -> ("error out"=w301:errorcluster)  [unwired: 7 in, 1 out]
        n179 = local write "Program State"("Check Max Torque" ("State")) -> ()
      }
      frame "Check Speed" {
        (unwired) "torque" ("Message")
        n180 = Unbundle By Name(w321) -> ("VISA resource name"=w317:refnum<visa-resource-name>)
        n181 = local read "Motor Status"() -> (w312:T1)
        n182 = for {
          N: 2 -> [_]
          tunnel: [w325] -> w315
          shift-right: [w329] -> w318
          shift-left: w319 -> [w330]
          shift-right: [w326] -> w316
          shift-left: w317 -> [w327]
          n183 = call "Read.vi"("error out"=w330, "Read"=T8 {"Index"="`ÿ", "Sub-Index"="\u0000", "Data-Size (in Byte)"=4, TRUE}, "ComPort In"=w327) -> ("error out 2"=w329:errorcluster, "Answer"=w325:i32, "ComPort Out"=w326:refnum<visa-resource-name>)  [unwired: 6 in]
          n184 = Wait (ms)(milliseconds to wait=u32 0) -> ()  [unwired: 1 out]
        }
        "error out" <- w318
        n185 = Unbundle By Name(w312) -> ("Motor Stopped"=w309:bool)  [unwired: 2 out]
        n186 = local write "Program State"("Checking Speed" ("State")) -> ()
        n187 = Bundle By Name(cluster=w321, "VISA resource name"=w316) -> (w320:T3)
        n188 = Select(t="Enable Voltage", s=w309, f="Wait" ("Message")) -> (s? t:f=w311:string)
        n189 = call-poly "Enqueue Message.vi"("error in (no error)"=w318, "Message"=w311, "Message Queue"=w322) -> ("error out"=w323:errorcluster)  [unwired: 7 in, 1 out]
        n190 = property on="Actual Speed RPM" class="Knob (strict)"("Value"=w315) -> ()  [unwired: 2 in, 2 out]
      }
      frame "Max Torque Change" {
        (unwired) "torque" ("Message")
        # "THIS IS REALLY INCORRECT AT THE MOMENT\nDO NOT TRUST ANY RESULTS FROM THIS EVENT CASE"
        # "Initialize - All initialization work should take place in this message, since other loops can potentially enqueue messages that execute immediately after this one."
        n191 = Unbundle By Name(w343) -> ("VISA resource name"=w338:refnum<visa-resource-name>)
        n192 = call "Read.vi"("error out"=w341, "Read"=T8 {"Index"=" 1", "Sub-Index"="\u0000", "Data-Size (in Byte)"=4, TRUE}, "ComPort In"=w338) -> ("error out 2"=w340:errorcluster, "Answer"=w336:i32, "ComPort Out"=w337:refnum<visa-resource-name>)  [unwired: 6 in]
        n193 = property on="Motor Initialized" class="Bool (strict)"() -> ("Value"=w333:bool)  [unwired: 2 in, 2 out]
        n194 = Bundle By Name(cluster=w343, "VISA resource name"=w337) -> (w342:T3)
        n195 = Select(t="Wait" ("Message"), s=w333, f="Halt Motor") -> (s? t:f=w332:string)
        n196 = call "Check Closed Loop.vi"("Answer"=w336) -> ("Bit 0"=w331:bool)  [unwired: 9 in, 1 out]
        n197 = call-poly "Enqueue Message.vi"("error in (no error)"=w340, "Message"=w332, "Message Queue"=w344) -> ("error out"=w345:errorcluster)  [unwired: 7 in, 1 out]
        n198 = property on="Closed Loop Available" class="Bool (strict)"("Value"=w331) -> ()  [unwired: 2 in, 2 out]
      }
      frame "Halt Motor" {
        w354 = "Check Closed Loop" ("Message")
        n199 = Unbundle By Name(w358) -> ("VISA resource name"=w353:refnum<visa-resource-name>)  [unwired: 1 out]
        n200 = property on="Read Torque" class="Bool (strict)"("Value"=FALSE ("Read Torque")) -> ()  [unwired: 2 in, 2 out]
        n201 = call "Fieldbus_Write_message.vi"("error in"=w347, "Message"="Halt") -> ("error output"=w346:errorcluster, "Write"=w351:T2)  [unwired: 8 in]
        n202 = local write "Motor Status"(T9 {"Motor Stopped"=FALSE, "Motor Running"=TRUE, "Motor Paused"=FALSE} ("Motor Status")) -> ()
        n203 = call "Write.vi"("error in"=w346, "Write"=w351, "ComPort In"=w353) -> ("error out"=w355:errorcluster, "ComPort Out"=w356:refnum<visa-resource-name>)  [unwired: 7 in]
        n204 = Bundle By Name(cluster=w358, "VISA resource name"=w356) -> (w357:T3)
        n205 = property on="Motor Initialized" class="Bool (strict)"("Value"=TRUE ("Motor Initialized")) -> ()  [unwired: 2 in, 2 out]
        n206 = call-poly "Enqueue Message.vi"("error in (no error)"=w355, "Message Data"=w354, "Message"=w354, "Message Queue"=w359) -> ("error out"=w360:errorcluster)  [unwired: 6 in, 1 out]
      }
      frame "Change Speed" {
        w371 = "Check Speed" ("Message")
        n207 = local read "Set Speed RPM"() -> (w362:i32)
        n208 = Unbundle By Name(w365) -> ("VISA resource name"=w370:refnum<visa-resource-name>)
        n209 = call "Fieldbus_Write_message.vi"("error in"=w361, "Data"=w362, "Message"="change speed") -> ("error output"=w364:errorcluster, "Write"=w368:T2)  [unwired: 7 in]
        "Write" <- w368
        n210 = property on="Apply Speed" class="Bool"("DisabledEnum"=T5."Disabled and Grayed Out" ("Disabled")) -> ()  [unwired: 2 in, 2 out]
        n211 = call "Write.vi"("error in"=w364, "Write"=w368, "ComPort In"=w370) -> ("error out"=w372:errorcluster, "ComPort Out"=w373:refnum<visa-resource-name>)  [unwired: 7 in]
        n212 = Bundle By Name(cluster=w365, "VISA resource name"=w373) -> (w374:T3)
        n213 = property on="User Event" class="Bool (strict)"("Value"=TRUE ("Doing Thing")) -> ()  [unwired: 2 in, 2 out]
        n214 = call-poly "Enqueue Message.vi"("error in (no error)"=w372, "Message Data"=w371, "Message"=w371, "Message Queue"=w363) -> ("error out"=w375:errorcluster)  [unwired: 6 in, 1 out]
      }
      frame "Speed Button" {
        # "Initialize - All initialization work should take place in this message, since other loops can potentially enqueue messages that execute immediately after this one."
        n215 = property on="Apply Speed" class="Bool"("DisabledEnum"=T5."Enabled" ("Disabled")) -> ()  [unwired: 2 in, 2 out]
        n216 = property on="User Event" class="Bool (strict)"("Value"=TRUE ("Doing Thing")) -> ()  [unwired: 2 in, 2 out]
        n217 = call-poly "Enqueue Message.vi"("error in (no error)"=w380, "Message"="Wait", "Message Queue"=w379) -> ("error out"=w377:errorcluster)  [unwired: 7 in, 1 out]
      }
      frame "Wait" {
        # "Initialize - All initialization work should take place in this message, since other loops can potentially enqueue messages that execute immediately after this one."
        n218 = local write "Program State"("Waiting" ("State")) -> ()
        n219 = property on="User Event" class="Bool (strict)"("Value"=FALSE ("Doing Thing")) -> ()  [unwired: 2 in, 2 out]
      }
      frame "Start Motor" {
        w393 = "Wait" ("Message")
        # "Initialize - All initialization work should take place in this message, since other loops can potentially enqueue messages that execute immediately after this one."
        n220 = Unbundle By Name(w397) -> ("VISA resource name"=w392:refnum<visa-resource-name>)
        n221 = call "Fieldbus_Write_message.vi"("error in"=w388, "Message"="Start") -> ("error output"=w387:errorcluster, "Write"=w390:T2)  [unwired: 8 in]
        n222 = call "Write.vi"("error in"=w387, "Write"=w390, "ComPort In"=w392) -> ("error out"=w394:errorcluster, "ComPort Out"=w395:refnum<visa-resource-name>)  [unwired: 7 in]
        n223 = local write "Motor Status"(T1 {"Motor Running"=TRUE, "Motor Paused"=FALSE, "Motor Stopped"=FALSE} ("Motor Status")) -> ()
        n224 = Bundle By Name(cluster=w397, "VISA resource name"=w395) -> (w396:T3)
        n225 = call-poly "Enqueue Message.vi"("error in (no error)"=w394, "Message Data"=w393, "Message"=w393, "Message Queue"=w398) -> ("error out"=w399:errorcluster)  [unwired: 6 in, 1 out]
      }
      frame "Get Torque" {
        (unwired) "torque" ("Message")
        # "Initialize - All initialization work should take place in this message, since other loops can potentially enqueue messages that execute immediately after this one."
        n226 = Unbundle By Name(w419) -> ("VISA resource name"=w414:refnum<visa-resource-name>)
        n227 = local read "Max Torque Nm"() -> (w405:dbl)
        n228 = local read "Max Motor Current mA"() -> (w406:dbl)
        n229 = local write "Program State"("Getting Torque from Motor" ("State")) -> ()
        n230 = call "Read.vi"("error out"=w417, "Read"=T8 {"Index"="`w", "Sub-Index"="\u0000", "Data-Size (in Byte)"=2, TRUE}, "ComPort In"=w414) -> ("error out 2"=w416:errorcluster, "Answer"=w412:i32, "ComPort Out"=w413:refnum<visa-resource-name>)  [unwired: 6 in]
        n231 = call "raw_torque_to_mA_and_kN.vi"("Max Motor Torque Nm"=w405, "Max Motor Current mA"=w406, "Torque % raw"=w412) -> ("Motor Torque Nm"=w404:dbl, "Motor Current mA"=w407:dbl, "Torque %"=w401:dbl)  [unwired: 6 in]
        n232 = Bundle By Name(cluster=w419, "VISA resource name"=w413) -> (w418:T3)
        n233 = Insert Into Array(array=w408, index=0, new element=w401) -> (w400:dbl[])
        n234 = call-poly "Enqueue Message.vi"("error in (no error)"=w416, "Message"="Get Torque", "Message Queue"=w420) -> ("error out"=w421:errorcluster)  [unwired: 7 in, 1 out]
        n235 = local write "Motor Current mA"(w407) -> ()
        n236 = call-poly <vilib>:"Butterworth Filter.vi"("init/cont (init:F)"=FALSE, "order"=2, "X"=w400) -> ()  [unwired: 5 in, 2 out]
        n237 = local write "Torque Nm"(w404) -> ()
        n238 = property on="Torque\n%" class="DigNum (strict)"("Value"=w401) -> ()  [unwired: 2 in, 2 out]
      }
      frame "Update Display" {
        # "#CodeRecommended - If you wish to decouple the Message Handling Loop from your user interface, consider creating User Events (like the \"Stop\" event in this VI) to message the Event Handling Loop whenever the user interface needs updating."
        # "Update Display - Convert the message data to a string to display in the Data Display indicator."
        n239 = Variant To Data(error in=w426, type="", Variant=w425) -> (data=w422:string, error out=w423:errorcluster)
        n240 = local write "Program State"(w422) -> ()
        n241 = Merge Errors(w423) -> (w427:errorcluster)
      }
      frame "Error" {
        # "#CodeRecommended - If you ever change the name of this \"Error\" message, you'll need to update the name in the Check Loop Error.vi as well."
        # "#CodeRecommended - Consider creating a system for logging errors in some way. These errors are for notification purposes only. Handling of specific errors should be performed in the message frames that generated the error."
        # "Error - Display an error dialog. This message is sent by the \"Error Handler\" VIs at the end of other loops in this application."
        n242 = Variant To Data(error in=w435, type=errorcluster {"status"=FALSE, "code"=0, "source"=""} ("error constant"), Variant=w433) -> (data=w431:errorcluster, error out=w430:errorcluster)
        n243 = call <vilib>:"Simple Error Handler.vi"("error in (no error)"=w431) -> ()  [unwired: 4 in, 5 out]
        n244 = Merge Errors(w430) -> (w429:errorcluster)
      }
      frame "Confirm Quit" {
        # "#CodeNeeded - If you want to provide an \"Are you sure\" dialog (or some other notification) before the application exits, place that code here. This message is typically sent from a Panel Close? event."
        # "Confirm Quit - Message that can confirm whether or not the user wants to exit the application."
        n245 = Unbundle By Name(w441) -> ("VISA resource name"=w445:refnum<visa-resource-name>)  [unwired: 1 out]
        n246 = call "Fieldbus_Write_message.vi"("error in"=w437, "Message"="Halt") -> ("error output"=w436:errorcluster, "Write"=w443:T2)  [unwired: 8 in]
        n247 = call "Write.vi"("error in"=w436, "Write"=w443, "ComPort In"=w445) -> ("error out"=w442:errorcluster, "ComPort Out"=w446:refnum<visa-resource-name>)  [unwired: 7 in]
        n248 = Bundle By Name(cluster=w441, "VISA resource name"=w446) -> (w440:T3)
        n249 = call-poly "Enqueue Message.vi"("Priority Message? (F)"=TRUE, "error in (no error)"=w437, "Message"="Exit", "Message Queue"=w449) -> ("error out"=w450:errorcluster)  [unwired: 6 in, 1 out]
        n250 = property on="Motor Initialized" class="Bool (strict)"("Value"=FALSE ("Motor Initialized")) -> ()  [unwired: 2 in, 2 out]
        n251 = local write "Motor Status"(T1 {"Motor Running"=FALSE, "Motor Paused"=FALSE, "Motor Stopped"=TRUE} ("Motor Status")) -> ()
        n252 = Merge Errors(w442, w450) -> (w451:errorcluster)
      }
      frame "Exit" {
        (unwired) ext 0.0 ("Numeric")
        (unwired) "0" ("String")
        # "Stop the VI"
        # "Release the message queue reference"
        # "#CodeNeeded - Add any required cleanup code here. Note that if 'Exit' was called as a result of an error, an error dialog will be displayed. Add any custom error handling for an 'Exit' condition here as well."
        # "Exit - Exit the application."
        n253 = Unbundle By Name(w457) -> ("VISA resource name"=w458:refnum<visa-resource-name>)
        n254 = Variant To Data(type=errorcluster {"status"=FALSE, "code"=0, "source"=""} ("error constant"), Variant=w459) -> (data=w460:errorcluster)  [unwired: 1 in, 1 out]
        n255 = call <vilib>:"Simple Error Handler.vi"("error in (no error)"=w460) -> ()  [unwired: 4 in, 5 out]
        n256 = VISA Close(VISA resource name=w458, error in (no error)=w456) -> (error out=w455:errorcluster)
        n257 = call "Fire User Event - Stop.vi"("User Event - Stop"=w463) -> ("error out"=w462:errorcluster)  [unwired: 10 in]
        n258 = Release Queue(queue=w467, error in (no error)=w455) -> (error out=w465:errorcluster)  [unwired: 1 in, 2 out]
        n259 = Merge Errors(w462, w465) -> (w464:errorcluster)
        n260 = local write "Motor Status"(T1 {"Motor Running"=FALSE, "Motor Paused"=FALSE, "Motor Stopped"=TRUE} ("Motor Status")) -> ()
        n261 = property on="Max Motor Current mA" class="DigNum (strict)"("Value"=0 ("Max Torque mA")) -> ()  [unwired: 2 in, 2 out]
        n262 = property on="Motor Initialized" class="Bool (strict)"("Value"=FALSE ("Motor Initialized")) -> ()  [unwired: 2 in, 2 out]
      }
      frame "Reinitialize Motor" {
        w474 = "Enable Voltage" ("Message")
        # "Initialize - All initialization work should take place in this message, since other loops can potentially enqueue messages that execute immediately after this one."
        n263 = Variant To Data(error in=w472, type=w473, Variant=w468) -> (data=w470:T3, error out=w471:errorcluster)
        n264 = Unbundle By Name(w470) -> ("VISA resource name"=w469:refnum<visa-resource-name>)
        n265 = VISA Open(error in (no error)=w471, VISA resource name=w469) -> (VISA resource name=w476:refnum<visa-resource-name>, error out=w475:errorcluster)  [unwired: 3 in]
        n266 = Bundle By Name(cluster=w473, "VISA resource name"=w476) -> (w477:T3)
        n267 = call-poly "Enqueue Message.vi"("error in (no error)"=w475, "Message Data"=w474, "Message"=w474, "Message Queue"=w478) -> ("error out"=w479:errorcluster)  [unwired: 6 in, 1 out]
      }
      frame Default {
        # "'Default' case only runs if there is a message that isn't defined in any of the other cases.  Output a programming error."
        n268 = xnode "Error Ring"("parameter 0"=w480) -> ("error out"=w481:errorcluster)
      }
    }
    "Torque % of Max" <- w111
    n269 = call "Error Handler - Message Handling Loop.vi"("error in (no error)"=w110, "Message Queue"=w113) -> ("dup error in"=w112:errorcluster)  [unwired: 8 in, 1 out]
  }
  n270 = Unregister For Events(event registration refnum=w9, error in=w7) -> (error out=w10:errorcluster)
  n271 = disable-structure shown="Disabled" {
    frame Disabled {
    }
    frame Enabled {
    }
  }
  n272 = Merge Errors(w10, w14) -> (w11:errorcluster)
  n273 = call "Destroy User Event - Stop.vi"("error in (no error)"=w11, "User Event - Stop"=w5) -> ("error out"=w8:errorcluster)  [unwired: 9 in]
  n274 = disable-structure shown="Default" {
    disable-tunnel: w8 -> [_ _]
    frame condition #0 (active) {
    }
    frame condition #1 {
      # "Call Quit LabVIEW if running as a built application."
      n275 = Quit LabVIEW() -> ()  [unwired: 1 in]
    }
  }
